vi "Set app state.vi"(3 "Error in":errorcluster, 4 "App state":T1) -> (0 "Error out":errorcluster)   [LabVIEW 2020]
uses:
  Global variables/Control and indicators refs.vi
  Typedefs/State.ctl
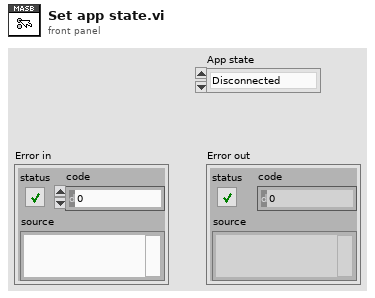
[diagram p1: front panel]
types:
  T1 = typedef "State.ctl" = enum16{"Disconnected", "Connected", "Measuring"}
  T2 = typedef "Control and indicators refs.ctl" = cluster{"Device":refnum<vi>, "Connect":refnum<vi>, "Measurement":refnum<vi>, "CV configuration":refnum<vi>, "I-V Graph":refnum<vi>}
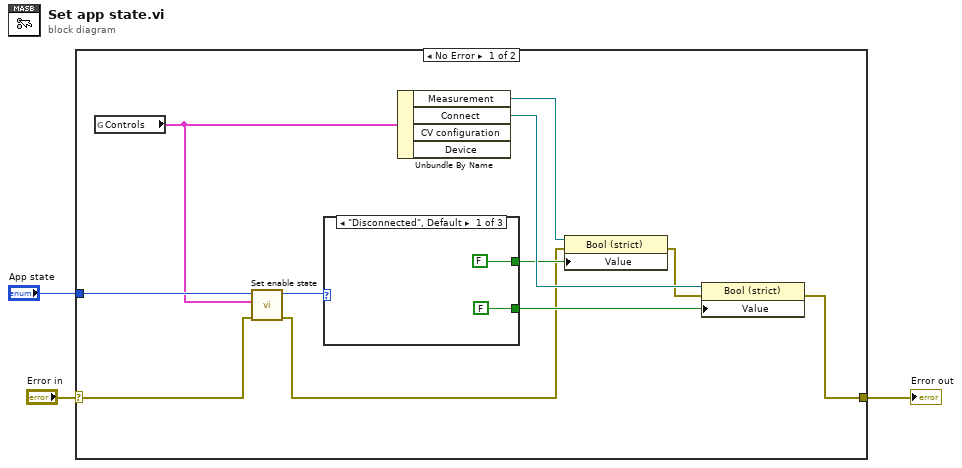
[diagram p0: block diagram]
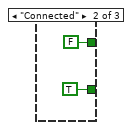
[diagram p2: hidden frame]
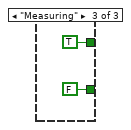
[diagram p3: hidden frame]
diagram:
  n1 = case shown="No Error" "Error in" {
    selector: "Error in" -> [w9 w21]
    tunnel: [w4 w21] -> w2
    tunnel: "App state" -> [w8 _]
    frame No Error {
      n2 = global read "Control and indicators refs.vi" "Controls"() -> (w7:T2)
      n3 = call "Set enable state.vi"("Error in"=w9, "Controls and indicators"=w7, "App state"=w8) -> ("Error out"=w5:errorcluster, "App state"=w6:T1)  [unwired: 7 in]
      n4 = case shown="\"Disconnected\", Default" w6 {
        tunnel: [FALSE FALSE TRUE] -> w11
        tunnel: [FALSE TRUE FALSE] -> w10
        frame "Disconnected", Default {
        }
        frame "Connected" {
        }
        frame "Measuring" {
        }
      }
      n5 = Unbundle By Name(w7) -> ("Measurement"=w14:refnum<vi>, "Connect"=w13:refnum<vi>)  [unwired: 2 out]
      n6 = property class="Bool (strict)"(reference=w14, error in=w5, "Value"=w11) -> (error out=w12:errorcluster)  [unwired: 1 out]
      n7 = property class="Bool (strict)"(reference=w13, error in=w12, "Value"=w10) -> (error out=w4:errorcluster)  [unwired: 1 out]
    }
    frame Error {
    }
  }
  "Error out" <- w2
